vi "PH_Watchdog.ProcEvents.vi"(0 "i ref in":refnum<vi>, 5 "error in (no error)":errorcluster) -> (14 "i ref out":refnum<vi>, 19 "error out":errorcluster)   [LabVIEW 2014, in "PH_Watchdog.lvlib"]
doc: "This method is used to define the events the object will listen to. Add your own events here."
uses:
  PH_Watchdog.lvlib
  CS_Core/BaseProcess/BaseProcess.lvlib
  PH_Basics/PH_Common/PH_Common.lvlib
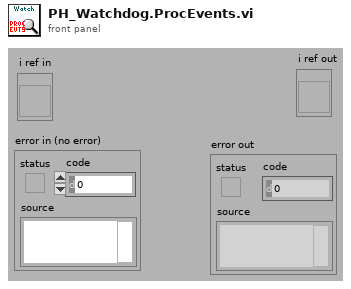
[diagram p1: front panel]
types:
  T1 = typedef "PH_Watchdog.lvlib/PH_Watchdog.i attribute.ctl" = cluster{"GUI Refs":cluster{"All":refnum<vi>, "Failures":refnum<vi>, "Alarms":refnum<vi>, "no info, but linked":refnum<vi>}, "All":T2[]}
  T2 = typedef "PH_Watchdog.lvlib/PH_Watchdog.Dataset.ctl" = cluster{"Instance":string, "Class":string, "Status":T3, "no Link":bool}
  T3 = typedef "PH_StatusHandler.lvlib/PH_StatusHandler.Status.ctl" = i16
  T4 = typedef "PH_Common.lvlib/PH_DIM.Event Declarer.ctl" = cluster{"Service Name":string, "Selector":string}
  T5 = typedef "BaseProcess.lvlib/BaseProcess.event definition.ctl" = cluster{"CAEEvtDef":T6, "Data Descriptor":T7}
  T6 = typedef "CAEObj.lvlib/CAEObj.event definition.ctl" = cluster{"URL":string, "enable":bool, "ignoreResID":bool}
  T7 = typedef "BaseProcess.lvlib/BaseProcess.descriptor string definition.ctl" = string
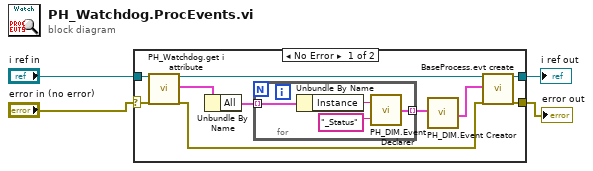
[diagram p0: block diagram]
diagram:
  n1 = case shown="No Error" "error in (no error)" {
    selector: "error in (no error)" -> [w12 w19]
    tunnel: "i ref in" -> [w11 w20]
    tunnel: [w14 w19] -> w3
    tunnel: [w13 w20] -> w2
    frame No Error {
      n2 = call "PH_Watchdog.get i attribute.vi"("i ref in"=w11, "error in (no error)"=w12) -> ("i ref out"=w10:refnum<vi>, "i attribute"=w8:T1, "error out"=w7:errorcluster)  [unwired: 15 in]
      n3 = Unbundle By Name(w8) -> ("All"=w6:T2[])
      n4 = for {
        tunnel: [w17] -> w5 mode=indexing
        tunnel: w6 -> [w16] mode=indexing
        n5 = Unbundle By Name(w16) -> ("Instance"=w15:string)
        n6 = call "PH_DIM.Event Declarer.vi"("Selector"="_Status", "Service Name"=w15) -> ("declared DIM Event"=w17:T4)
      }
      n7 = call "PH_DIM.Event Creator.vi"("Status Services"=w5) -> ("DIM Service Events"=w9:T5[])  [unwired: 18 in]
      n8 = call "BaseProcess.evt create.vi"("i ref in"=w10, "newEvents"=w9, "error in (no error)"=w7) -> ("i ref out"=w13:refnum<vi>, "error out"=w14:errorcluster)  [unwired: 13 in, 2 out]
    }
    frame Error {
    }
  }
  "i ref out" <- w2
  "error out" <- w3
